vi "Day4_Template.vi"() -> ()   [LabVIEW 2026]
uses:
  <vilib>/numeric/Random Number (Range) U64.vi
  <vilib>/numeric/sub_Random U32.vi
panel:
  in  "Mode":enum32{"Simulated", "Hardware"}(radio)
  in  "Stop":bool
  in  "Buttons":bool[](array[boolean])
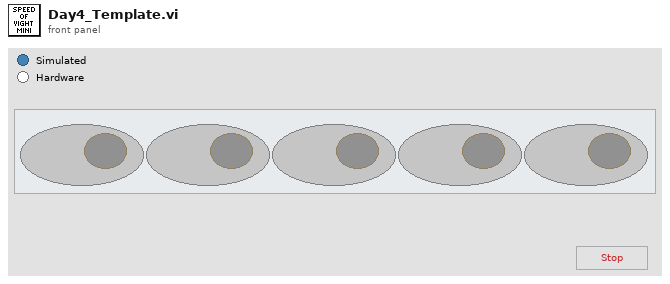
[diagram p1: front panel]
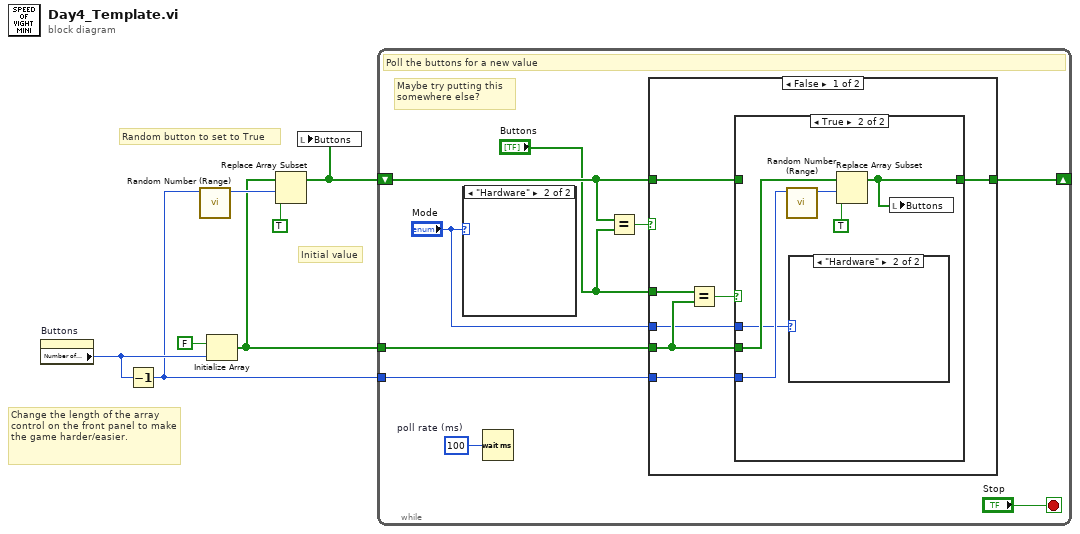
[diagram p0: block diagram]
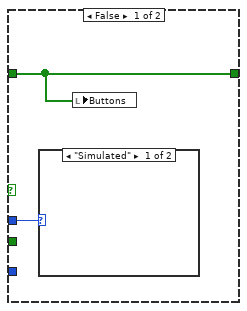
[diagram p2: hidden frame]
diagram:
  # "Random button to set to True"
  # "Initial value"
  # "Change the length of the array control on the front panel to make the game harder/easier."
  n1 = property on="Buttons" class="Arr (strict)"() -> ("Number of Columns"=w2:u32)  [unwired: 2 in, 2 out]
  n2 = Decrement(x=w2) -> (x-1=w1:u32)
  n3 = call-poly <vilib>:"Random Number (Range).vi"("upper bound (100)"=w1) -> ("number"=w6:u64)  [unwired: 10 in]
  n4 = Initialize Array(FALSE, w2) -> (w5:bool[])
  n5 = Replace Array Subset(array=w5, new element=TRUE ("new element/subarray"), index=w6) -> (w3:bool[])
  n6 = local write "Buttons"(w3) -> ()
  n7 = while {
    tunnel: w5 -> [w11]
    shift-right: [w12] -> _
    shift-left: w3 -> [w13]
    tunnel: w1 -> [w10]
    stop <- "Stop" stop-if-true
    w15 = u32 100  # poll rate (ms)
    # "Maybe try putting this\nsomewhere else?"
    # "Poll the buttons for a new value"
    n8 = case shown="\"Hardware\"" "Mode" {
      frame "Simulated" {
      }
      frame "Hardware" {
      }
    }
    n9 = Wait (ms)(milliseconds to wait=w15) -> ()  [unwired: 1 out]
    n10 = Equal?(x=w13, y="Buttons") -> (x = y?=w14:bool)
    n11 = case shown="False" w14 {
      tunnel: w13 -> [w18 w32]
      tunnel: [w20 w32] -> w12
      tunnel: w11 -> [w19 _]
      tunnel: "Buttons" -> [w23 _]
      tunnel: w10 -> [w21 _]
      tunnel: "Mode" -> [w17 _]
      frame False {
        # "Button value changed, see if they clicked the correct button."
        n12 = Equal?(x=w23, y=w19) -> (x = y?=w22:bool)
        n13 = case shown="True" w22 {
          tunnel: w21 -> [_ w28]
          tunnel: [w25 w27] -> w20
          tunnel: w19 -> [_ w29]
          tunnel: w18 -> [w25 _]
          tunnel: w17 -> [w24 w26]
          frame False {
            # "Wrong button clicked. Decrement score and un-click button."
            n14 = case shown="\"Simulated\"" w24 {
              frame "Simulated" {
              }
              frame "Hardware" {
                # "In hardware mode you'll need a way to send the new value to the hardware to turn on/off button lights appropriately."
              }
            }
            n15 = local write "Buttons"(w25) -> ()
          }
          frame True {
            # "Correct button clicked, update score and set a new random value"
            n16 = call-poly <vilib>:"Random Number (Range).vi"("upper bound (100)"=w28) -> ("number"=w30:u64)  [unwired: 10 in]
            n17 = case shown="\"Hardware\"" w26 {
              frame "Simulated" {
              }
              frame "Hardware" {
              }
            }
            n18 = Replace Array Subset(array=w29, new element=TRUE ("new element/subarray"), index=w30) -> (w27:bool[])
            n19 = local write "Buttons"(w27) -> ()
          }
        }
      }
      frame True {
        # "Button value did not change"
      }
    }
  }
